vi "readFromXML.vi"(8 "error in (no error)":errorcluster, 10 "XML in":string, 11 "ClearCollOffset in":refnum<class "ClearCollOffset.lvclass">) -> (0 "error out":errorcluster, 3 "ClearCollOffset out":refnum<class "ClearCollOffset.lvclass">)   [LabVIEW 2022 SP3, in "TCSDataDefinitions.lvlib" / "TCSCommand.lvlib" / "OffsetCommands.lvlib" / "ClearCollOffset.lvclass"]
uses:
  ClearCollOffset.lvclass
  CollimationOffsetCommands/CollimationOffsetCommands.lvclass
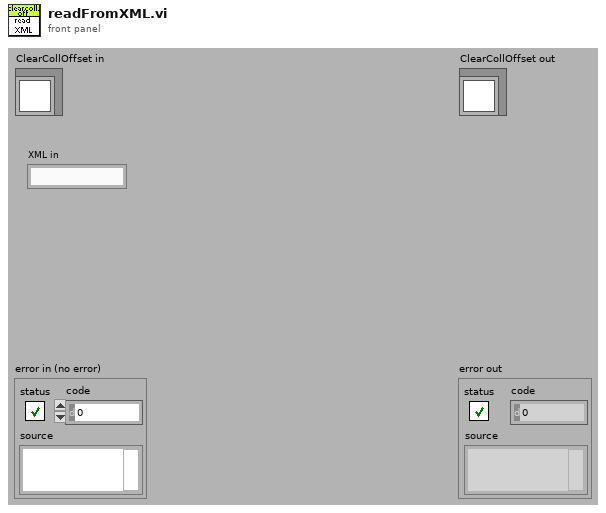
[diagram p1: front panel]
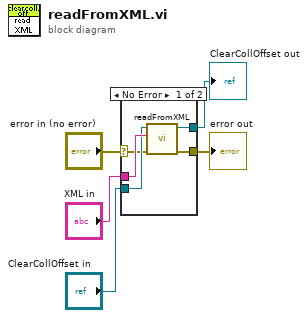
[diagram p0: block diagram]
diagram:
  n1 = case shown="No Error" "error in (no error)" {
    selector: "error in (no error)" -> [w6 w11]
    tunnel: [w10 w11] -> w5
    tunnel: [w9 w12] -> w4
    tunnel: "XML in" -> [w8 _]
    tunnel: "ClearCollOffset in" -> [w7 w12]
    frame No Error {
      n2 = call-parent "readFromXML.vi"("error in (no error)"=w6, "XML in"=w8, "CollimationOffsetCommands in"=w7) -> ("error out"=w10:errorcluster, "CollimationOffsetCommands out"=w9:refnum<class "ClearCollOffset.lvclass">)  [unwired: 7 out]
    }
    frame Error {
    }
  }
  "error out" <- w5
  "ClearCollOffset out" <- w4
